vi "Integrator (DBL).vi"(2 "initialize":bool, 3 "dt":dbl=1e-09 min=1e-09 format="%.6f", 4 "initial condition":dbl format="%.2f", 5 "input point":dbl format="%.2f") -> (1 "output point":dbl format="%.2f")   [LabVIEW 2017, in "NI_AdvCtrl_continuous linear.lvlib"]
doc: "LabVIEW no longer supports this VI. You can obtain similar functionality by installing the LabVIEW Simulation Module.\n\nIntegrates a continuous input signal. The integration process is based on Euler method. dt must be positive."
uses:
  <vilib>/addons/control/advanced/NI_AdvCtrl_continuous linear.lvlib
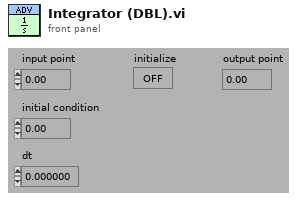
[diagram p1: front panel]
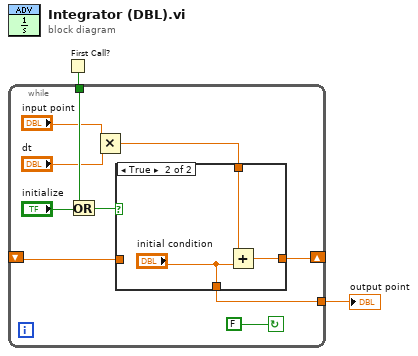
[diagram p0: block diagram]
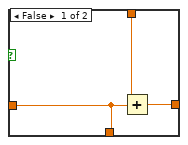
[diagram p2: hidden frame]
diagram:
  n1 = First Call?() -> (First Call?: T/F=w2:bool)
  n2 = while {
    tunnel: [w3] -> w1
    tunnel: w2 -> [w9]
    shift-left: _ -> [w4]
    shift-right: [w12] -> _
    stop <- FALSE continue-if-true
    n3 = Or(x=w9, y="initialize") -> (x .or. y?=w8:bool)
    n4 = Multiply(x="input point", y="dt") -> (x*y=w6:dbl)
    n5 = case shown="True" w8 {
      tunnel: [w15 w18] -> w12
      tunnel: w4 -> [w13 _]
      tunnel: w6 -> [w14 w17]
      tunnel: [w13 "initial condition"] -> w3
      frame False {
        n6 = Add(x=w14, y=w13) -> (x+y=w15:dbl)
      }
      frame True {
        n7 = Add(x=w17, y="initial condition") -> (x+y=w18:dbl)
      }
    }
  }
  "output point" <- w1
